vi "Hub.vi"() -> ()   [LabVIEW 2017]
panel:
  in  "ON/OFF":bool
  out "Smoke Alarm":bool
  out "Gas Alarm":bool
  out "Heater On":bool
  out "Cooler On":bool
  out "Smoke Sys On":bool
  out "Temp Sys On":bool
  out "Gas Sys On":bool
  # "Smart Hub"
  # "Illo inc."
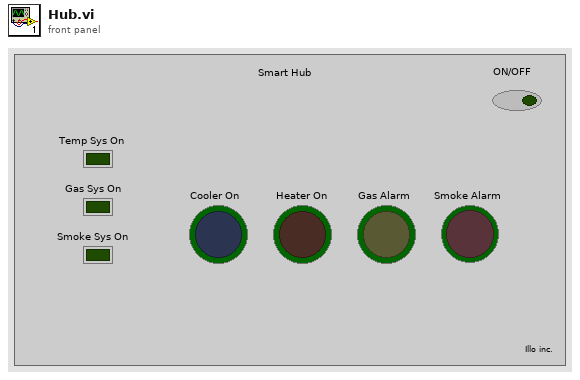
[diagram p1: front panel]
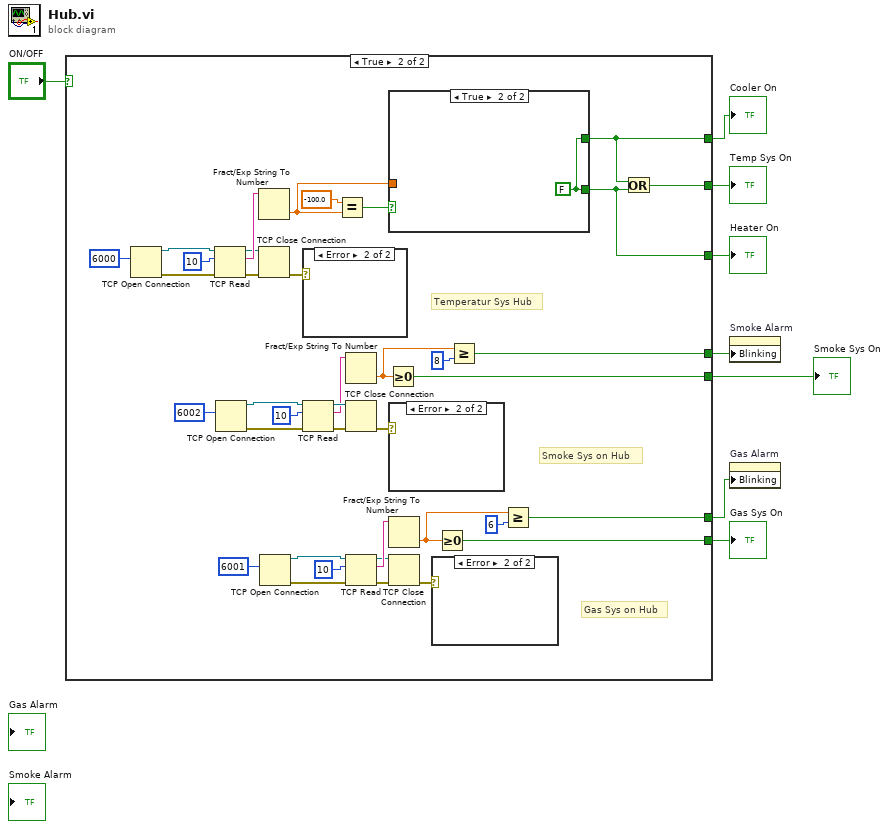
[diagram p0: block diagram]
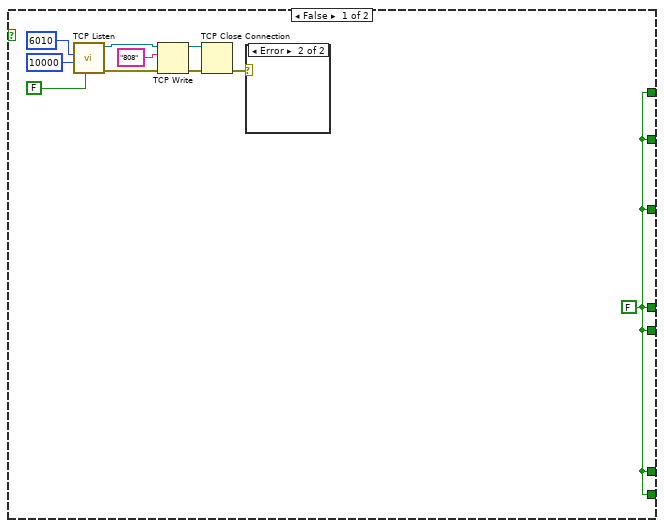
[diagram p2: hidden frame]
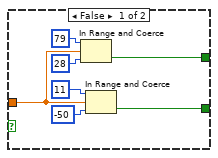
[diagram p4: hidden frame]
diagram:
  n1 = case shown="True" "ON/OFF" {
    tunnel: [w18 w28] -> w7
    tunnel: [w18 w27] -> w6
    tunnel: [w18 w26] -> w5
    tunnel: [w18 w25] -> w4
    tunnel: [w18 w24] -> w3
    tunnel: [w18 w23] -> w2
    tunnel: [w18 w22] -> w1
    frame False {
      w18 = FALSE
      n2 = call <vilib>:"TCP Listen.vi"("resolve remote address (T)"=FALSE, "timeout ms (wait forever: -1)"=10000, "port"=6010) -> ("error out"=w16:errorcluster, "connection ID"=w14:refnum<k5>)  [unwired: 4 in, 3 out]
      n3 = TCP Write(connection ID=w14, data in="808", error in (no error)=w16) -> (connection ID out=w13:refnum<k5>, error out=w15:errorcluster)  [unwired: 1 in, 1 out]
      n4 = TCP Close Connection(connection ID=w13, error in (no error)=w15) -> (error out=w10:errorcluster)  [unwired: 1 in, 1 out]
      n5 = case shown="Error" w10 {
        frame No Error {
        }
        frame Error {
        }
      }
    }
    frame True {
      # "Smoke Sys on Hub"
      # "Gas Sys on Hub"
      # "Temperatur Sys Hub"
      n6 = TCP Open Connection(remote port or service name=6000) -> (connection ID=w38:refnum<k5>, error out=w37:errorcluster)  [unwired: 4 in]
      n7 = TCP Read(connection ID=w38, bytes to read=10, error in (no error)=w37) -> (connection ID out=w40:refnum<k5>, data out=w41:string, error out=w39:errorcluster)  [unwired: 2 in]
      n8 = TCP Open Connection(remote port or service name=6002) -> (connection ID=w49:refnum<k5>, error out=w48:errorcluster)  [unwired: 4 in]
      n9 = Fract/Exp String To Number(string=w41) -> (number=w20:dbl)  [unwired: 3 in, 1 out]
      n10 = TCP Close Connection(connection ID=w40, error in (no error)=w39) -> (error out=w42:errorcluster)  [unwired: 1 in, 1 out]
      n11 = TCP Open Connection(remote port or service name=6001) -> (connection ID=w44:refnum<k5>, error out=w43:errorcluster)  [unwired: 4 in]
      n12 = case shown="Error" w42 {
        frame No Error {
        }
        frame Error {
        }
      }
      n13 = TCP Read(connection ID=w49, bytes to read=10, error in (no error)=w48) -> (connection ID out=w52:refnum<k5>, data out=w51:string, error out=w50:errorcluster)  [unwired: 2 in]
      n14 = Equal?(x=-100.0, y=w20) -> (x = y?=w21:bool)
      n15 = Fract/Exp String To Number(string=w51) -> (number=w56:dbl)  [unwired: 3 in, 1 out]
      n16 = TCP Close Connection(connection ID=w52, error in (no error)=w50) -> (error out=w53:errorcluster)  [unwired: 1 in, 1 out]
      n17 = TCP Read(connection ID=w44, bytes to read=10, error in (no error)=w43) -> (connection ID out=w46:refnum<k5>, data out=w47:string, error out=w45:errorcluster)  [unwired: 2 in]
      n18 = Greater Or Equal To 0?(x=w56) -> (x >= 0?=w23:bool)
      n19 = case shown="True" w21 {
        tunnel: w20 -> [w63 _]
        tunnel: [w58 w64] -> w25
        tunnel: [w57 w64] -> w24
        frame False {
          n20 = In Range and Coerce(upper limit=79, x=w63, lower limit=28) -> (In Range?=w57:bool)  [unwired: 1 out]
          n21 = In Range and Coerce(upper limit=11, x=w63, lower limit=-50) -> (In Range?=w58:bool)  [unwired: 1 out]
        }
        frame True {
          w64 = FALSE
        }
      }
      n22 = case shown="Error" w53 {
        frame No Error {
        }
        frame Error {
        }
      }
      n23 = Fract/Exp String To Number(string=w47) -> (number=w55:dbl)  [unwired: 3 in, 1 out]
      n24 = TCP Close Connection(connection ID=w46, error in (no error)=w45) -> (error out=w54:errorcluster)  [unwired: 1 in, 1 out]
      n25 = case shown="Error" w54 {
        frame No Error {
        }
        frame Error {
        }
      }
      n26 = Greater Or Equal To 0?(x=w55) -> (x >= 0?=w22:bool)
      n27 = Greater Or Equal?(x=w56, y=8) -> (x >= y?=w27:bool)
      n28 = Greater Or Equal?(x=w55, y=6) -> (x >= y?=w28:bool)
      n29 = Or(x=w24, y=w25) -> (x .or. y?=w26:bool)
    }
  }
  "Temp Sys On" <- w5
  "Heater On" <- w4
  "Cooler On" <- w3
  "Smoke Sys On" <- w2
  "Gas Sys On" <- w1
  n30 = property on="Smoke Alarm" class="Bool (strict)"("Blinking"=w6) -> ()  [unwired: 2 in, 2 out]
  n31 = property on="Gas Alarm" class="Bool (strict)"("Blinking"=w7) -> ()  [unwired: 2 in, 2 out]
